vi "get_rois.vi"(8 "Error In":errorcluster, 10 "Sample":string, 11 "File Path":path) -> (0 "Error Out":errorcluster)   [LabVIEW 2019]
uses:
  grain_results_cluster_typedef.ctl
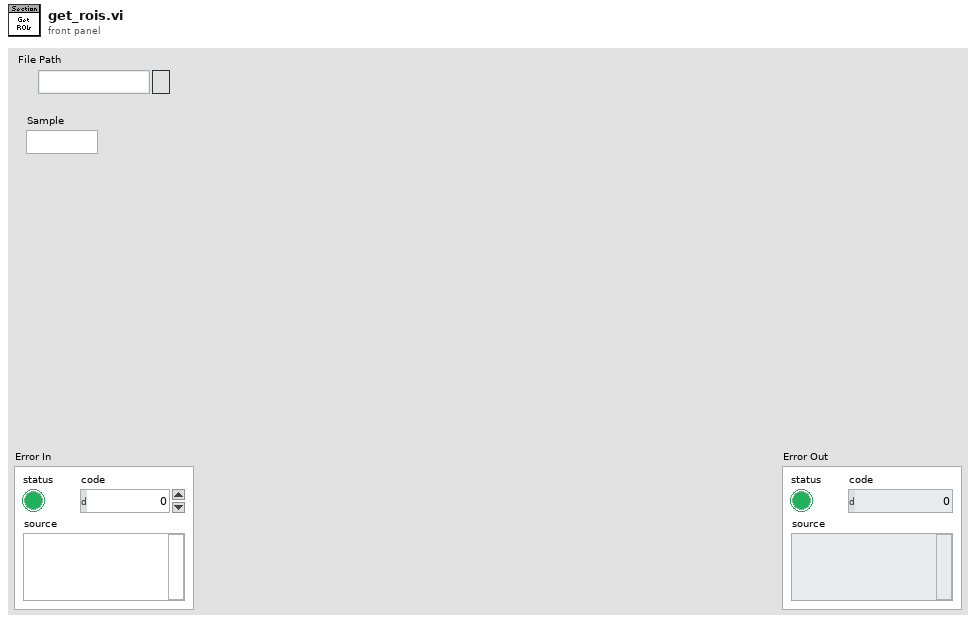
[diagram p1: front panel]
types:
  T1 = typedef "grain_results_cluster_typedef.ctl" = cluster{"Grain Number":i32, "xi":dbl[], "phiin":dbl[], "Intensity":dbl[][], "Best Fit Intensity":dbl[][], "Best Fit Parameters":dbl[][], "Polarizer 1 Angle":dbl[][], "Polarizer 2 Angle":dbl[][], "Best Extinction Angle":dbl[], "Best Extinction Angle Corrected":dbl[], "Thetac":dbl, "Phic":dbl, "ROI":cluster{"Global Rectangle":i32[], "Contours":cluster{"Contour Type":u32, "ROI Type":u32, "Points":i32[]}[]}, "a":dbl, "b":dbl, "sequences available":dbl, "sequences used":dbl, "Contrast":dbl[], "Rsq":dbl}
  T2 = cluster{"Global Rectangle":i32[], "Contours":cluster{"Contour Type":u32, "ROI Type":u32, "Points":i32[]}[]}[]
  T3 = typedef "sample_results_cluster_typedef.ctl" = cluster{"File Path":string, "Sample":string, "Threshold":dbl, "Parameters":T4, "Writeable Parameters":T5, "Gain Results":T1[]}
  T4 = typedef "parameters_cluster_typedef.ctl" = cluster{"m1":dbl, "m2":dbl, "m3":dbl, "c":dbl, "D":dbl, "Beta":dbl, "center x":dbl, "center y":dbl}
  T5 = typedef "writeable_section_parameters_cluster_typedef.ctl" = cluster{"Section":string, "Method":i32, "Edge Mode":i32, "Grid Constant":i32, "Manual Sequence":i32, "ROI Size":i32, "Min Grain Size":dbl, "Comments":string, "File Path":string}
  T6 = typedef "section_parameters_cluster_typedef.ctl" = cluster{"Section":string, "Method":T7, "Edge Mode":T8, "ROI Size":T9, "Manual Sequence":T10, "Grid Constant":i32, "Min Grain Size":dbl, "Comments":string, "File Path":path}
  T7 = typedef "sections_method_enum_typedef.ctl" = enum16{"Edge Detection", "Grid Only", "Manual Selection", "Existing Edges"}
  T8 = typedef "sections_edge_mode_enum_typedef.ctl" = enum16{"Grid for Large Grains Only", "Grid", "No Grid"}
  T9 = typedef "sections_roi_size_enum_typedef.ctl" = enum16{"0x0", "1x1", "2x2", "3x3", "4x4", "5x5", "6x6"}
  T10 = typedef "xi_angles_enum_typedef.ctl" = enum16{"0", "45"}
  T11 = cluster{"Global Rectangle":i32[], "Contours":cluster{"ID":enum32{"External", "Internal"}, "Type":enum32{"No Selection", "Point", "Line", "Rectangle", "Oval", "Polygon", "Free", "Unused1", "Unused2", "Unused3", "Broken Line", "Free Hand Line"}, "Coordinates":i32[]}[]}[]
  T12 = cluster{"Global Rectangle":i32[], "Contours":cluster{"Contour Type":u32, "ROI Type":u32, "Points":i32[]}[]}
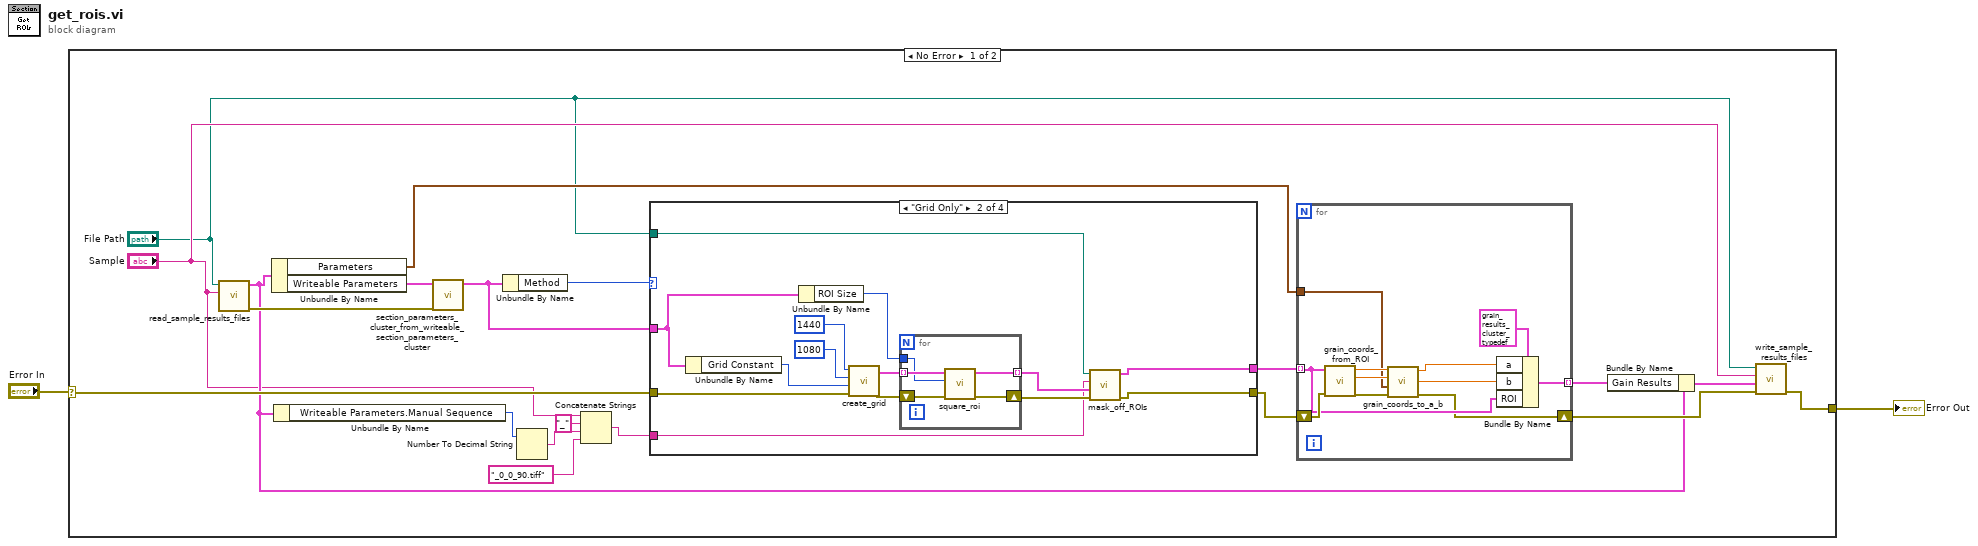
[diagram p0: block diagram]
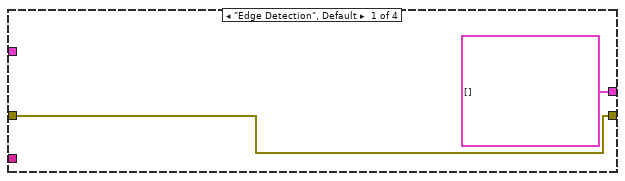
[diagram p2: hidden frame]
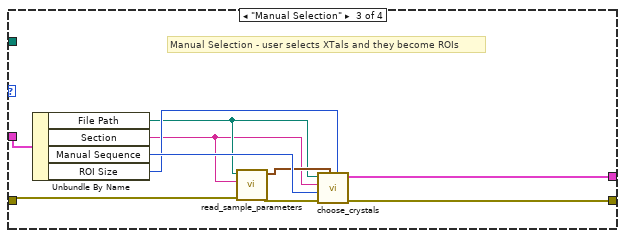
[diagram p3: hidden frame]
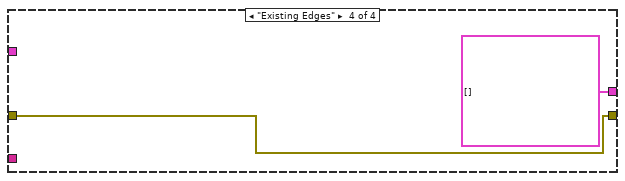
[diagram p4: hidden frame]
diagram:
  n1 = case shown="No Error" "Error In" {
    selector: "Error In" -> [w12 w67]
    tunnel: [w11 w67] -> w1
    frame No Error {
      n2 = call "read_sample_results_files.vi"("Sample"="Sample", "File Path"="File Path") -> ("Error Out"=w19:errorcluster, "Sample Results"=w10:T3)  [unwired: 8 in]
      n3 = Unbundle By Name(w10) -> ("Parameters"=w16:T4, "Writeable Parameters"=w21:T5)
      n4 = Unbundle By Name(w10) -> ("Writeable Parameters.Manual Sequence"=w8:i32)
      n5 = call "section_parameters_cluster_from_writeable_section_parameters_cluster.vi"("Error In"=w19, "Writeable Parameters"=w21) -> ("Section Parameters"=w20:T6)  [unwired: 8 in, 1 out]
      n6 = Unbundle By Name(w20) -> ("Method"=w22:T7)
      n7 = Number To Decimal String(number=w8) -> (decimal integer string=w7:string)  [unwired: 1 in]
      n8 = Concatenate Strings("Sample", "_" ("string"), w7, "_0_0_90.tiff" ("string")) -> (w4:string)
      n9 = case shown="\"Grid Only\"" w22 {
        tunnel: w20 -> [_ w44 w64 _]
        tunnel: w12 -> [w34 w47 w57 w65]
        tunnel: [T2 [] ("ROIs Out") w39 w56 T2 [] ("ROIs Out")] -> w18
        tunnel: [w34 w40 w55 w65] -> w17
        tunnel: w4 -> [_ w37 _ _]
        tunnel: "File Path" -> [_ w36 _ _]
        frame "Edge Detection", Default {
        }
        frame "Grid Only" {
          n10 = Unbundle By Name(w44) -> ("Grid Constant"=w46:i32)
          n11 = Unbundle By Name(w44) -> ("ROI Size"=w43:T9)
          n12 = call "create_grid.vi"("Error In"=w47, "Grid Constant"=w46, "Y Size"=1080, "X Size"=1440) -> ("Error Out"=w42:errorcluster, "Array"=w45:T11)  [unwired: 6 in]
          n13 = for {
            tunnel: w45 -> [w54] mode=indexing
            tunnel: w43 -> [w53]
            shift-right: [w51] -> w41
            shift-left: w42 -> [w52]
            tunnel: [w50] -> w38 mode=indexing
            n14 = call "square_roi.vi"("Error In"=w52, "ROI Size"=w53, "ROI In"=w54) -> ("Error Out"=w51:errorcluster, "ROI Out"=w50:T12)  [unwired: 7 in]
          }
          n15 = call "mask_off_ROIs.vi"("Error In"=w41, "ROIs In"=w38, "Image Name"=w37, "Path"=w36) -> ("Error Out"=w40:errorcluster, "ROIs out"=w39:T2)  [unwired: 6 in]
        }
        frame "Manual Selection" {
          # "Manual Selection - user selects XTals and they become ROIs"
          n16 = Unbundle By Name(w64) -> ("File Path"=w59:path, "Section"=w58:string, "Manual Sequence"=w63:T10, "ROI Size"=w62:T9)
          n17 = call "read_sample_parameters.vi"("Error In"=w57, "Sample"=w58, "File Path"=w59) -> ("Error Out"=w60:errorcluster, "Parameters"=w61:T4)  [unwired: 6 in, 1 out]
          n18 = call "choose_crystals.vi"("ROI Size"=w62, "Parameters"=w61, "Error In"=w60, "Xi"=w63, "Sample"=w58, "File Path"=w59) -> ("Error Out"=w55:errorcluster, "ROIs Out"=w56:T2)  [unwired: 4 in]
        }
        frame "Existing Edges" {
        }
      }
      n19 = for {
        tunnel: w18 -> [w25] mode=indexing
        tunnel: w16 -> [w29]
        tunnel: [w24] -> w15 mode=indexing
        shift-right: [w23] -> w13
        shift-left: w17 -> [w33]
        n20 = call "grain_coords_from_ROI.vi"("Error In"=w33, "ROI In"=w25) -> ("Error Out"=w30:errorcluster, "y"=w31:dbl, "x"=w32:dbl)  [unwired: 7 in]
        n21 = call "grain_coords_to_a_b.vi"("Error In"=w30, "Parameters"=w29, "y"=w31, "x"=w32) -> ("Error Out"=w23:errorcluster, "b"=w26:dbl, "a"=w27:dbl)  [unwired: 5 in]
        n22 = Bundle By Name(cluster=T1 {"Grain Number"=0, "xi"=[], "phiin"=[], "Intensity"=[], "Best Fit Intensity"=[], "Best Fit Parameters"=[], "Polarizer 1 Angle"=[], "Polarizer 2 Angle"=[], "Best Extinction Angle"=[], "Best Extinction Angle Corrected"=[], "Thetac"=0.0, "Phic"=0.0, "ROI"={"Global Rectangle"=[], "Contours"=[]}, "a"=0.0, "b"=0.0, "sequences available"=0.0, "sequences used"=0.0, "Contrast"=[], "Rsq"=0.0} ("Grain Results"), "a"=w27, "b"=w26, "ROI"=w25) -> (w24:T1)
      }
      n23 = Bundle By Name(cluster=w10, "Gain Results"=w15) -> (w14:T3)
      n24 = call "write_sample_results_files.vi"("Error In"=w13, "Sample Results"=w14, "Sample"="Sample", "File Path"="File Path") -> ("Error Out"=w11:errorcluster)  [unwired: 7 in]
    }
    frame Error {
    }
  }
  "Error Out" <- w1
